vi "FYP_VI_MIDI_Data.vi"(1 "MIDI Channel":u32, 2 "Mode On / Off":u32, 3 "Pitch Note":u32, 4 "Velocity / Volume":u32) -> (0 "MIDI data":u32)   [LabVIEW 2013]
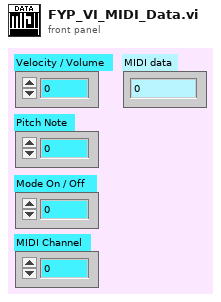
[diagram p1: front panel]
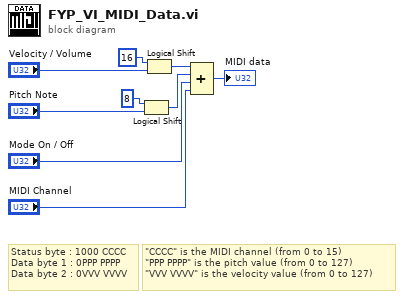
[diagram p0: block diagram]
diagram:
  # "\"CCCC\" is the MIDI channel (from 0 to 15)\n\"PPP PPPP\" is the pitch value (from 0 to 127)\n\"VVV VVVV\" is the velocity value (from 0 to 127)"
  # "Status byte : 1000 CCCC\nData byte 1 : 0PPP PPPP\nData byte 2 : 0VVV VVVV"
  n1 = Logical Shift(y=i16 8, x="Pitch Note") -> (x << y=w4:u32)
  n2 = Logical Shift(y=i16 16, x="Velocity / Volume") -> (x << y=w5:u32)
  n3 = Compound Arithmetic op=ADD(w5, w4, "Mode On / Off", "MIDI Channel") -> (→"MIDI data":u32)
